vi "kloehn_test.vi"() -> ()   [LabVIEW 2010]
panel:
  out "error out":errorcluster
  # "This VI is just a simple test of the Kloehn system. It should open a session, initialize the device (run Init Kloehn), then run inject sample, then finally close out the session."
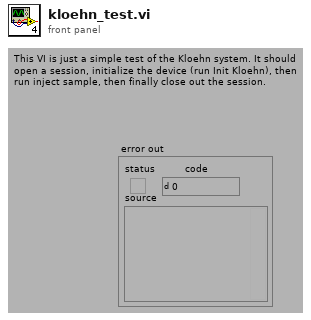
[diagram p1: front panel]
types:
  T1 = cluster{"baud rate (9600)":u32, "data bits (8)":u16, "parity (0:none)":enum16{"None", "Odd", "Even", "Mark", "Space"}, "stop bits (10: 1 bit)":u16, "flow control (0:none)":u16, "timeout (10sec)":u32, "termination char\n(0xA = '\\n' = LF) ":u8, "Enable Termination\nChar (T)":bool}
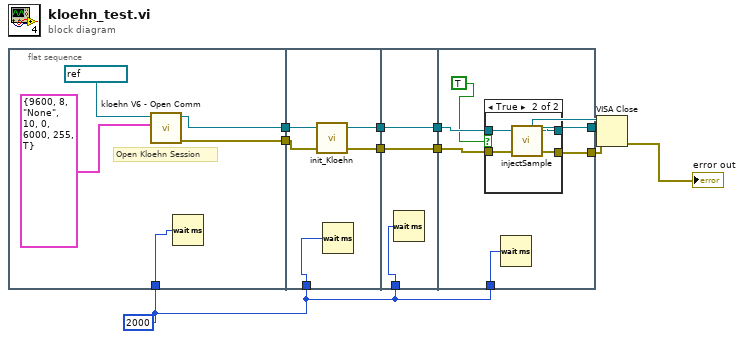
[diagram p0: block diagram]
diagram:
  w1 = 2000
  n1 = flat-sequence {
    tunnel: [w13] -> w10
    tunnel: [w12] -> w9
    tunnel: w1 -> [w11]
    tunnel: w10 -> [w20]
    tunnel: w9 -> [w19]
    tunnel: [w18] -> w5
    tunnel: [w17] -> w3
    tunnel: w1 -> [w16]
    tunnel: w5 -> [w23]
    tunnel: [w23] -> w4
    tunnel: w3 -> [w22]
    tunnel: [w22] -> w2
    tunnel: w1 -> [w21]
    tunnel: w4 -> [w28]
    tunnel: w2 -> [w29]
    tunnel: [w27] -> w8
    tunnel: [w26] -> w7
    tunnel: w1 -> [w25]
    frame #0 {
      # "Open Kloehn Session"
      n2 = call "kloehn V6 - Open Comm .vi"("Serial Parameters"=T1 {"baud rate (9600)"=9600, "data bits (8)"=8, "parity (0:none)"=enum."None", "stop bits (10: 1 bit)"=10, "flow control (0:none)"=0, "timeout (10sec)"=6000, "termination char\n(0xA = '\\n' = LF) "=255, "Enable Termination\nChar (T)"=TRUE} ("Port Configuration"), "VISA Ref in"=refnum<visa-resource-name> "COM10" ("Koehn VISA Ref")) -> ("error out"=w12:errorcluster, "VISA Ref out"=w13:refnum<visa-resource-name>)  [unwired: 8 in]
      n3 = Wait (ms)(milliseconds to wait=w11) -> ()  [unwired: 1 out]
    }
    frame #1 {
      n4 = call "init_Kloehn.vi"("error in"=w19, "VISA resource in"=w20) -> ("error out"=w17:errorcluster, "VISA resource out"=w18:refnum<visa-resource-name>)  [unwired: 2 in]
      n5 = Wait (ms)(milliseconds to wait=w16) -> ()  [unwired: 1 out]
    }
    frame #2 {
      n6 = Wait (ms)(milliseconds to wait=w21) -> ()  [unwired: 1 out]
    }
    frame #3 {
      n7 = case shown="True" TRUE {
        tunnel: w29 -> [w30 w35]
        tunnel: w28 -> [w31 w34]
        tunnel: [w31 w33] -> w27
        tunnel: [w30 w32] -> w26
        frame False {
        }
        frame True {
          n8 = call "injectSample.vi"("error in"=w35, "VISA resource in"=w34) -> ("error out"=w32:errorcluster, "VISA resource out"=w33:refnum<visa-resource-name>)  [unwired: 2 in]
        }
      }
      n9 = Wait (ms)(milliseconds to wait=w25) -> ()  [unwired: 1 out]
    }
  }
  n10 = VISA Close(VISA resource name=w8, error in (no error)=w7) -> (error out=→"error out":errorcluster)
